vi "checkRules.vi"(8 "error in (no error)":errorcluster, 10 "tcp packet":string, 11 "tcpServer in":refnum<class "TcpServer.lvclass">) -> (0 "error out":errorcluster, 2 "is ok?":bool, 3 "tcpServer out":refnum<class "TcpServer.lvclass">)   [LabVIEW 2018, in "TcpServer.lvclass"]
doc: "Check command rules to allow command to be sent to User."
uses:
  TcpServer.lvclass
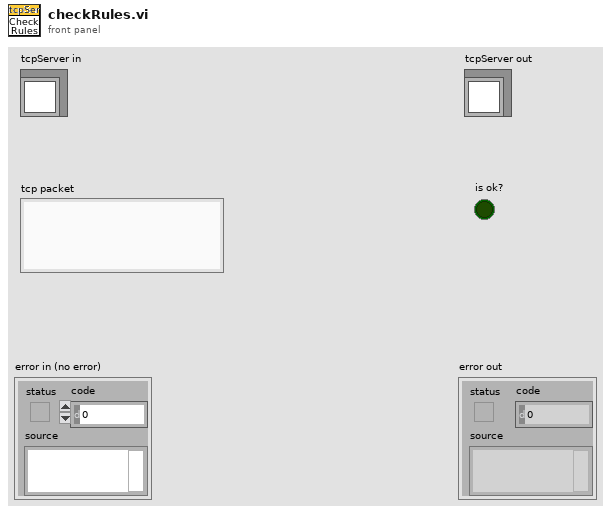
[diagram p1: front panel]
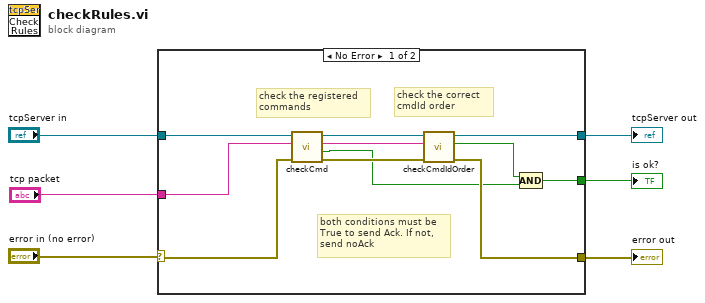
[diagram p0: block diagram]
diagram:
  n1 = case shown="No Error" "error in (no error)" {
    selector: "error in (no error)" -> [w17 w19]
    tunnel: [w10 w19] -> w5
    tunnel: [w13 w18] -> w3
    tunnel: "tcpServer in" -> [w16 w18]
    tunnel: "tcp packet" -> [w9 _]
    tunnel: [w15 _] -> w1
    frame No Error {
      # "both conditions must be\nTrue to send Ack. If not,\nsend noAck"
      # "check the correct \ncmdId order"
      # "check the registered\ncommands"
      n2 = call "checkCmd.vi"("error in (no error)"=w17, "tcp packet"=w9, "tcpServer in"=w16) -> ("error out"=w11:errorcluster, "allowed?"=w7:bool, "tcp packet out"=w8:string, "tcpServer out"=w14:refnum<class "TcpServer.lvclass">)  [unwired: 5 in]
      n3 = call "checkCmdIdOrder.vi"("error in (no error)"=w11, "json command"=w8, "tcpServer in"=w14) -> ("error out"=w10:errorcluster, "ok"=w12:bool, "tcpServer out"=w13:refnum<class "TcpServer.lvclass">)  [unwired: 6 in]
      n4 = Compound Arithmetic op=AND(w12, w7) -> (w15:bool)
    }
    frame Error {
    }
  }
  "error out" <- w5
  "tcpServer out" <- w3
  "is ok?" <- w1
